vi "Start Server.vi"(5 "Server Key File (.key)":path, 7 "Server Certificate File (.crt)":path, 8 "error in":errorcluster, 10 "gRPCid server in":T1, 11 "Server Address":string) -> (0 "error out":errorcluster, 2 "Listening Port":i32, 3 "gRPCid server out":T1)   [LabVIEW 2019, in "grpc-lvsupport.lvlib"]
uses:
  grpc-lvsupport.lvlib
  Shared/grpcId.ctl
  <vilib>/Utility/error.llb/Error Cluster From Error Code.vi
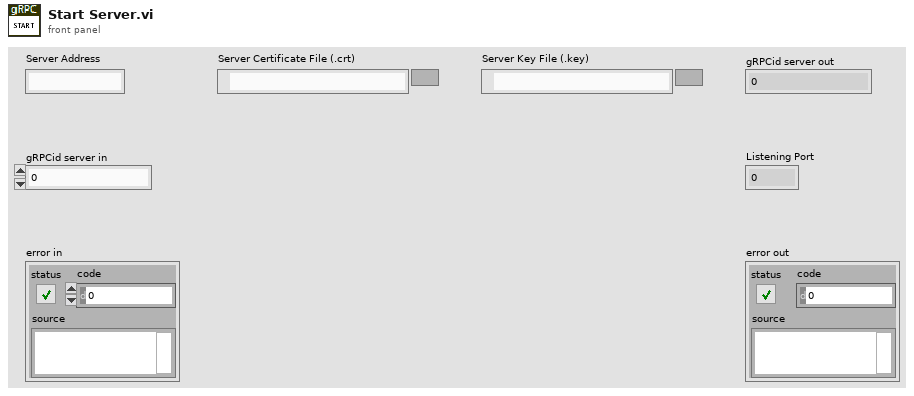
[diagram p1: front panel]
types:
  T1 = typedef "grpc-lvsupport.lvlib/grpcId.ctl" = u64
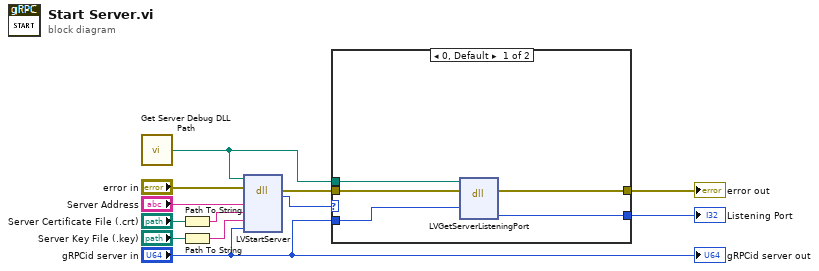
[diagram p0: block diagram]
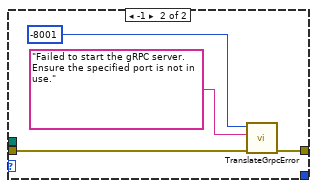
[diagram p2: hidden frame]
diagram:
  n1 = call "Get Server Debug DLL Path.vi"() -> ("Server dll path"=w4:path)
  n2 = Path To String(path="Server Certificate File (.crt)") -> (string=w9:string)
  n3 = Path To String(path="Server Key File (.key)") -> (string=w8:string)
  n4 = dll-call lib="?" fn="LVStartServer"(path in=w4, error in="error in", "serveraddress"="Server Address", "serverCertificateFile"=w9, "serverKeyFile"=w8, "serverid"="gRPCid server in") -> (error out=w11:errorcluster, "return type"=w5:i32)  [unwired: 5 in, 1 out]
  n5 = case shown="0, Default" w5 {
    tunnel: [w17 w18] -> w2
    tunnel: w11 -> [w16 w21]
    tunnel: w4 -> [w15 _]
    tunnel: "gRPCid server in" -> [w14 _]
    tunnel: [w13 _] -> w1
    frame 0, Default {
      n6 = dll-call lib="?" fn="LVGetServerListeningPort"(path in=w15, error in=w16, "serverId"=w14) -> (error out=w17:errorcluster, "listeningPort"=w13:i32)  [unwired: 4 in, 1 out]
    }
    frame -1 {
      n7 = call "TranslateGrpcError.vi"("error in"=w21, "Error Message"="Failed to start the gRPC server.  Ensure the specified port is not in use.", "Error Code"=-8001) -> ("error out"=w18:errorcluster)  [unwired: 8 in]
    }
  }
  "error out" <- w2
  "Listening Port" <- w1
  "gRPCid server out" <- "gRPCid server in"
